vi "Begin.vi"(11 "Image Size":T1=enum."160x120") -> (0 "error out":errorcluster)   [LabVIEW 2012]
doc: "Called before other user functions, this VI is expected to open initial I/O refnums, load in file data, and do all program initialization. Notice that the <B>error out</B> terminal is simply used for data flow. Wiring it to other structures or subVIs ensures that this VI runs first."
uses:
  <vilib>/Rock Robotics/WPI/Camera/WPI_CameraImageSize.ctl
  <vilib>/Rock Robotics/WPI/Camera/WPI_CameraWhite Balance Values.ctl
  <vilib>/Rock Robotics/WPI/Camera/WPI_CameraExposure Values.ctl
  <vilib>/Rock Robotics/WPI/Camera/WPI_CameraFrameRate.ctl
  <vilib>/Rock Robotics/WPI/DriverStation/WPI_DriverStationRobotMode2.ctl
  <vilib>/Rock Robotics/SystemInterfaces/DIO/FPGA_DIOChannel.ctl
  <vilib>/Rock Robotics/SystemInterfaces/AI/FPGA_AIGyroChannel.ctl
  <vilib>/Rock Robotics/WPI/Relay/WPI_RelayDirection.ctl
  <vilib>/Rock Robotics/SystemInterfaces/DIO/FPGA_DIORelayChannel.ctl
  <vilib>/Rock Robotics/SystemInterfaces/DIO/FPGA_DIOPWMChannel.ctl
  <vilib>/Rock Robotics/SystemInterfaces/Typedef/FPGA_TypedefDigitalModule.ctl
  <vilib>/Rock Robotics/WPI/Joystick/WPI_JoystickDeviceEnum.ctl
  <vilib>/Rock Robotics/SystemInterfaces/AI/FPGA_AIChannel.ctl
  Robot Global Data.vi
  <vilib>/Rock Robotics/WPI/MotorControl/WPI_MotorControlOpen Victor.vi
  <vilib>/Rock Robotics/WPI/MotorControl/WPI_MotorControlOpen Jaguar.vi
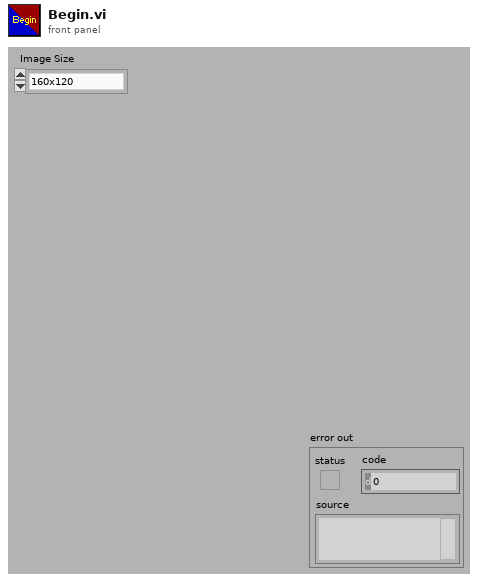
[diagram p1: front panel]
types:
  T1 = typedef "WPI_CameraImageSize.ctl" = enum16{"640x480", "320x240", "160x120"}
  T2 = typedef "FPGA_AIChannel.ctl" = enum8{"AI 1", "AI 2", "AI 3", "AI 4", "AI 5", "AI 6", "AI 7", "AI 8", "Invalid"}
  T3 = typedef "FPGA_TypedefDigitalModule.ctl" = enum16{"Digital Module 1", "Digital Module 2"}
  T4 = typedef "FPGA_DIOPWMChannel.ctl" = enum8{"PWM 1", "PWM 2", "PWM 3", "PWM 4", "PWM 5", "PWM 6", "PWM 7", "PWM 8", "PWM 9", "PWM 10", "Invalid"}
  T5 = typedef "WPI_JoystickDeviceEnum.ctl" = enum16{"USB 1", "USB 2", "USB 3", "USB 4", "Kinect 1", "Kinect 2"}
  T6 = typedef "FPGA_DIORelayChannel.ctl" = enum8{"Relay 1", "Relay 2", "Relay 3", "Relay 4", "Relay 5", "Relay 6", "Relay 7", "Relay 8", "Invalid"}
  T7 = typedef "WPI_RelayDirection.ctl" = enum16{"Both directions", "Forward only", "Reverse only"}
  T8 = typedef "FPGA_AIGyroChannel.ctl" = enum8{"AI 1", "AI 2", "Invalid"}
  T9 = typedef "FPGA_DIOChannel.ctl" = enum8{"DIO 1", "DIO 2", "DIO 3", "DIO 4", "DIO 5", "DIO 6", "DIO 7", "DIO 8", "DIO 9", "DIO 10", "DIO 11", "DIO 12", "DIO 13", "DIO 14", "Invalid"}
  T10 = typedef "WPI_DriverStationRobotMode2.ctl" = enum16{"Autonomous Disabled", "Autonomous Enabled", "Teleop Disabled", "Teleop Enabled", "Timeout", "Finish", "Test Disabled", "Test Enabled"}
  T11 = typedef "WPI_CameraFrameRate.ctl" = u32
  T12 = typedef "WPI_CameraExposure Values.ctl" = enum16{"Auto", "Flicker-free 50 Hz", "Flicker-free 60 Hz", "Hold current"}
  T13 = typedef "WPI_CameraWhite Balance Values.ctl" = enum16{"Auto", "Fixed indoor", "Fixed outdoor 1", "Fixed outdoor 2", "Fixed fluorescent 1", "Fixed fluorescent 2", "Hold current"}
  T14 = typedef "WPI_ServoDeviceRef.ctl" = cluster{"DeviceStatus":errorcluster, "Digital Module":T3, "PWM Channel":T4, "DeadBand":T15}
  T15 = typedef "WPI_PWMDeadband.ctl" = cluster{"Name":string, "maxPositivePwm":i32, "minPositivePwm":i32, "centerPwm":i32, "maxNegativePwm":i32, "minNegativePwm":i32, "angularRange":u16}
  T16 = typedef "WPI_CameraDevRef.ctl" = cluster{"Camera Address":string, "CameraStatus":errorcluster, "Acquire Image Notifier":refnum<notifier>}
  T17 = typedef "WPI_MotorControlDeviceRef.ctl" = cluster{"DeviceStatus":errorcluster, "Type":enum16{"PWM", "CAN"}, "PWM":cluster{"Digital Module":T3, "PWM Channel":T4, "DeadBand":T15}, "CAN":cluster{"Device Number":u8, "Control Mode":T18, "Semaphore":T19, "Max Vout":dbl}, "Invert":bool, "TransformRef":T20, "InvTransformRef":T20}
  T18 = typedef "WPI_CANJaguar_ControlMode.ctl" = enum8{"Percent VBus", "Current", "Speed", "Position", "Voltage"}
  T19 = typedef "Semaphore RefNum" = refnum<k1>
  T20 = typedef "WPI_PWMTransform_ConPane.ctl" = refnum<vi>
  T21 = typedef "WPI_JoystickDevRef.ctl" = cluster{"Device":T5}
  T22 = typedef "WPI_AnalogChannelDevRef.ctl" = cluster{"DevStatus":errorcluster, "Analog Module":T23, "Analog Channel":T2}
  T23 = typedef "FPGA_TypedefAnalogModule.ctl" = enum16{"Analog Module 1", "Analog Module 2"}
  T24 = typedef "WPI_RelayDevRef.ctl" = cluster{"DevStatus":errorcluster, "Relay Channel":T6, "Digital Module":T3, "Relay Direction":T7}
  T25 = typedef "WPI_DigitalInputDevRef.ctl" = cluster{"DevStatus":errorcluster, "DIO Channel":T9, "Digital Module":T3}
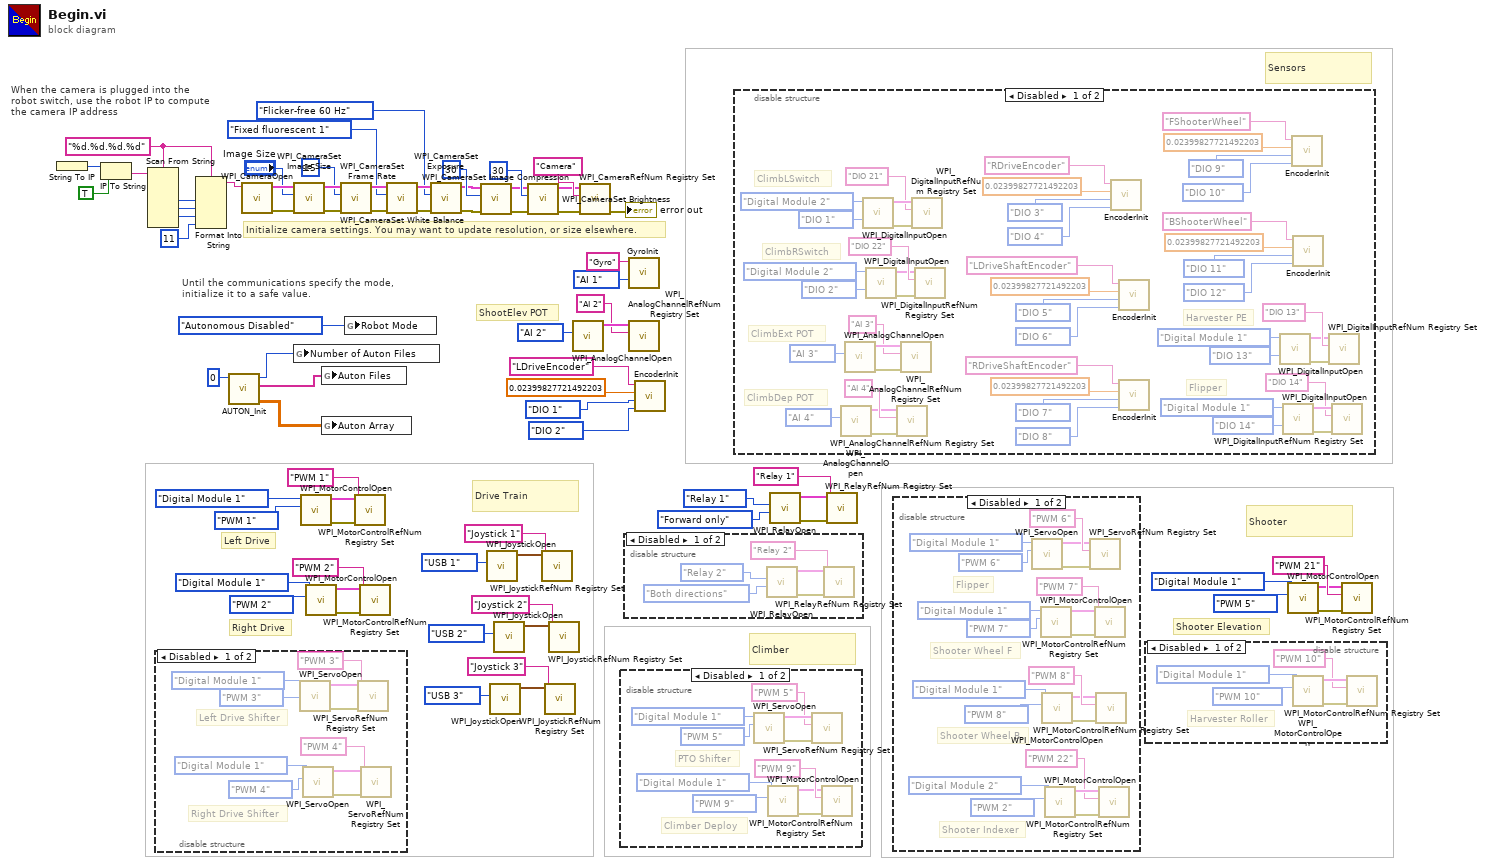
[diagram p0: block diagram]
diagram:
  w46 = "%d.%d.%d.%d" ("format string")
  # "ShootElev POT"
  # "Drive Train"
  # "Climber"
  # "Shooter"
  # "Shooter Elevation"
  # "Sensors"
  # "Right Drive"
  # "Left Drive"
  # "Until the communications specify the mode,\ninitialize it to a safe value."
  # "When the camera is plugged into the\nrobot switch, use the robot IP to compute\nthe camera IP address"
  # "Initialize camera settings. You may want to update resolution, or size elsewhere."
  n1 = String To IP() -> (0:w53:u32)  [unwired: 1 in]
  n2 = IP To String(1:TRUE ("dot notation? (F)"), 2:w53) -> (0:w51:string)
  n3 = Scan From String(format string=w46, input string=w51) -> (output 1=w50:i32, output 2=w49:i32, output 3=w48:i32)  [unwired: 7 in, 3 out]
  n4 = disable-structure shown="Disabled" {
    frame Disabled {
      # "Right Drive Shifter"
      # "Left Drive Shifter"
      n5 = call <vilib>:"WPI_ServoOpen.vi"("PWM Channel"=FPGA_DIOPWMChannel."PWM 3", "Digital Module (Module 1)"=FPGA_TypedefDigitalModule."Digital Module 1") -> ("error out"=w76:errorcluster, "ServoDeviceRef"=w77:T14)  [unwired: 8 in]
      n6 = call <vilib>:"WPI_ServoOpen.vi"("PWM Channel"=FPGA_DIOPWMChannel."PWM 4", "Digital Module (Module 1)"=FPGA_TypedefDigitalModule."Digital Module 1") -> ("error out"=w75:errorcluster, "ServoDeviceRef"=w82:T14)  [unwired: 8 in]
      n7 = call <vilib>:"WPI_ServoRefNum Registry Set.vi"("error in (no error)"=w76, "refnum name"="PWM 3", "ServoDeviceRef"=w77) -> ()  [unwired: 7 in, 2 out]
      n8 = call <vilib>:"WPI_ServoRefNum Registry Set.vi"("error in (no error)"=w75, "refnum name"="PWM 4", "ServoDeviceRef"=w82) -> ()  [unwired: 7 in, 2 out]
    }
    frame Enabled {
    }
  }
  n9 = Format Into String(format string=w46, w50, w49, w48, 11 ("Compression")) -> (resulting string=w44:string)  [unwired: 2 in, 1 out]
  n10 = call "AUTON_Init.vi"("Default File"=0) -> ("Auton Array"=w39:dbl[][], "Auton Files"=w40:string[], "Number of Auton Files"=w41:i64)  [unwired: 8 in]
  n11 = call <vilib>:"WPI_CameraOpen.vi"("Camera Address"=w44) -> ("error out"=w65:errorcluster, "CameraDevRef"=w66:T16)  [unwired: 1 in, 8 out]
  n12 = call <vilib>:"WPI_CameraSet Image Size.vi"("error in (no error)"=w65, "Image Size"="Image Size", "CameraDevRef"=w66) -> ("error out"=w64:errorcluster, "CameraDevRef Out"=w67:T16)  [unwired: 7 out]
  n13 = global write "Robot Global Data.vi" "Number of Auton Files"(w41) -> ()
  n14 = call-poly <vilib>:"WPI_MotorControlOpen.vi"("PWM Channel"=FPGA_DIOPWMChannel."PWM 1", "Digital Module (Module 1)"=FPGA_TypedefDigitalModule."Digital Module 1") -> ("error out"=w18:errorcluster, "MotorControlDeviceRef"=w19:T17)  [unwired: 8 in]
  n15 = call-poly <vilib>:"WPI_MotorControlOpen.vi"("PWM Channel"=FPGA_DIOPWMChannel."PWM 2", "Digital Module (Module 1)"=FPGA_TypedefDigitalModule."Digital Module 1") -> ("error out"=w25:errorcluster, "MotorControlDeviceRef"=w24:T17)  [unwired: 8 in]
  n16 = global write "Robot Global Data.vi" "Auton Files"(w40) -> ()
  n17 = global write "Robot Global Data.vi" "Auton Array"(w39) -> ()
  n18 = call <vilib>:"WPI_CameraSet Frame Rate.vi"("error in (no error)"=w64, "Frame Rate (fps)"=T11 15, "CameraDevRef"=w67) -> ("error out"=w63:errorcluster, "CameraDevRef Out"=w69:T16)  [unwired: 7 out]
  n19 = global write "Robot Global Data.vi" "Robot Mode"(WPI_DriverStationRobotMode2."Autonomous Disabled" ("Robot Mode")) -> ()
  n20 = call <vilib>:"WPI_MotorControlRefNum Registry Set.vi"("error in (no error)"=w18, "refnum name"="PWM 1", "MotorControlDevRef"=w19) -> ()  [unwired: 7 in, 2 out]
  n21 = call <vilib>:"WPI_MotorControlRefNum Registry Set.vi"("error in (no error)"=w25, "refnum name"="PWM 2", "MotorControlDevRef"=w24) -> ()  [unwired: 7 in, 2 out]
  n22 = call <vilib>:"WPI_CameraSet White Balance.vi"("error in (no error)"=w63, "White Balance"=WPI_CameraWhite_Balance_Values."Fixed fluorescent 1", "CameraDevRef"=w69) -> ("error out"=w62:errorcluster, "CameraDevRef Out"=w68:T16)  [unwired: 7 out]
  n23 = call <vilib>:"WPI_CameraSet Exposure.vi"("error in (no error)"=w62, "Exposure"=WPI_CameraExposure_Values."Flicker-free 60 Hz", "CameraDevRef"=w68) -> ("error out"=w61:errorcluster, "CameraDevRef Out"=w71:T16)  [unwired: 7 out]
  n24 = call <vilib>:"WPI_CameraSet Image Compression.vi"("error in (no error)"=w61, "Compression"=30, "CameraDevRef"=w71) -> ("error out"=w60:errorcluster, "CameraDevRef Out"=w70:T16)  [unwired: 7 out]
  n25 = call <vilib>:"WPI_JoystickOpen.vi"("JoystickDevice"=WPI_JoystickDeviceEnum."USB 1") -> ("JoystickDevRef"=w9:T21)  [unwired: 10 in]
  n26 = call <vilib>:"WPI_JoystickOpen.vi"("JoystickDevice"=WPI_JoystickDeviceEnum."USB 3") -> ("JoystickDevRef"=w15:T21)  [unwired: 10 in]
  n27 = call <vilib>:"WPI_JoystickOpen.vi"("JoystickDevice"=WPI_JoystickDeviceEnum."USB 2") -> ("JoystickDevRef"=w14:T21)  [unwired: 10 in]
  n28 = call <vilib>:"WPI_CameraSet Brightness.vi"("error in (no error)"=w60, "Brightness"=30, "CameraDevRef"=w70) -> ("error out"=w58:errorcluster, "CameraDevRef Out"=w59:T16)  [unwired: 7 out]
  n29 = call <vilib>:"WPI_JoystickRefNum Registry Set.vi"("refnum name"="Joystick 1", "JoystickDevRef"=w9) -> ()  [unwired: 8 in, 2 out]
  n30 = call <vilib>:"WPI_JoystickRefNum Registry Set.vi"("refnum name"="Joystick 3", "JoystickDevRef"=w15) -> ()  [unwired: 8 in, 2 out]
  n31 = call <vilib>:"WPI_JoystickRefNum Registry Set.vi"("refnum name"="Joystick 2", "JoystickDevRef"=w14) -> ()  [unwired: 8 in, 2 out]
  n32 = call <vilib>:"WPI_AnalogChannelOpen.vi"("Analog Channel"=FPGA_AIChannel."AI 2") -> ("AIDeviceRef"=w3:T22)  [unwired: 9 in, 1 out]
  n33 = call <vilib>:"WPI_CameraRefNum Registry Set.vi"("error in (no error)"=w58, "refnum name"="Camera", "CameraDevRef"=w59) -> ("error out"=→"error out":errorcluster)  [unwired: 8 out]
  n34 = disable-structure shown="Disabled" {
    frame Disabled {
      # "Climber Deploy"
      # "PTO Shifter"
      n35 = call <vilib>:"WPI_ServoOpen.vi"("PWM Channel"=FPGA_DIOPWMChannel."PWM 5", "Digital Module (Module 1)"=FPGA_TypedefDigitalModule."Digital Module 1") -> ("error out"=w94:errorcluster, "ServoDeviceRef"=w93:T14)  [unwired: 8 in]
      n36 = call-poly <vilib>:"WPI_MotorControlOpen.vi"("PWM Channel"=FPGA_DIOPWMChannel."PWM 9", "Digital Module (Module 1)"=FPGA_TypedefDigitalModule."Digital Module 1") -> ("error out"=w88:errorcluster, "MotorControlDeviceRef"=w87:T17)  [unwired: 8 in]
      n37 = call <vilib>:"WPI_ServoRefNum Registry Set.vi"("error in (no error)"=w94, "refnum name"="PWM 5", "ServoDeviceRef"=w93) -> ()  [unwired: 7 in, 2 out]
      n38 = call <vilib>:"WPI_MotorControlRefNum Registry Set.vi"("error in (no error)"=w88, "refnum name"="PWM 9", "MotorControlDevRef"=w87) -> ()  [unwired: 7 in, 2 out]
    }
    frame Enabled {
    }
  }
  n39 = disable-structure shown="Disabled" {
    frame Disabled {
      n40 = call <vilib>:"WPI_RelayOpen.vi"("Relay Direction"=WPI_RelayDirection."Both directions", "Relay Channel"=FPGA_DIORelayChannel."Relay 2") -> ("error out"=w95:errorcluster, "RelayDevRef"=w96:T24)  [unwired: 8 in]
      n41 = call <vilib>:"WPI_RelayRefNum Registry Set.vi"("error in (no error)"=w95, "refnum name"="Relay 2", "RelayDevRef"=w96) -> ()  [unwired: 7 in, 2 out]
    }
    frame Enabled {
    }
  }
  n42 = call "GyroInit.vi"("refnum name"="Gyro", "Analog Channel"=FPGA_AIGyroChannel."AI 1") -> ()  [unwired: 8 in]
  n43 = call <vilib>:"WPI_AnalogChannelRefNum Registry Set.vi"("refnum name"="AI 2", "AIDeviceRef"=w3) -> ()  [unwired: 8 in, 2 out]
  n44 = call "EncoderInit.vi"("refnum name"="LDriveEncoder", "DistancePerCount"=0.02399827721492203, "DIO Channel"=FPGA_DIOChannel."DIO 1", "DIO Channel 2"=FPGA_DIOChannel."DIO 2") -> ()  [unwired: 7 in]
  n45 = disable-structure shown="Disabled" {
    frame Disabled {
      # "ClimbRSwitch"
      # "ClimbLSwitch"
      # "ClimbDep POT"
      # "ClimbExt POT"
      # "Flipper"
      # "Harvester PE"
      n46 = call <vilib>:"WPI_AnalogChannelOpen.vi"("Analog Channel"=FPGA_AIChannel."AI 4") -> ("error out"=w114:errorcluster, "AIDeviceRef"=w115:T22)  [unwired: 9 in]
      n47 = call <vilib>:"WPI_AnalogChannelOpen.vi"("Analog Channel"=FPGA_AIChannel."AI 3") -> ("error out"=w113:errorcluster, "AIDeviceRef"=w112:T22)  [unwired: 9 in]
      n48 = call <vilib>:"WPI_DigitalInputOpen.vi"("DIO Channel"=FPGA_DIOChannel."DIO 1", "Digital Module (Module 1)"=FPGA_TypedefDigitalModule."Digital Module 2") -> ("error out"=w101:errorcluster, "DigitalInputDevRef"=w102:T25)  [unwired: 8 in]
      n49 = call <vilib>:"WPI_DigitalInputOpen.vi"("DIO Channel"=FPGA_DIOChannel."DIO 2", "Digital Module (Module 1)"=FPGA_TypedefDigitalModule."Digital Module 2") -> ("error out"=w108:errorcluster, "DigitalInputDevRef"=w107:T25)  [unwired: 8 in]
      n50 = call <vilib>:"WPI_AnalogChannelRefNum Registry Set.vi"("error in (no error)"=w114, "refnum name"="AI 4", "AIDeviceRef"=w115) -> ()  [unwired: 7 in, 2 out]
      n51 = call <vilib>:"WPI_AnalogChannelRefNum Registry Set.vi"("error in (no error)"=w113, "refnum name"="AI 3", "AIDeviceRef"=w112) -> ()  [unwired: 7 in, 2 out]
      n52 = call <vilib>:"WPI_DigitalInputRefNum Registry Set.vi"("error in (no error)"=w101, "refnum name"="DIO 21", "DigitalInputDevRef"=w102) -> ()  [unwired: 7 in, 2 out]
      n53 = call <vilib>:"WPI_DigitalInputRefNum Registry Set.vi"("error in (no error)"=w108, "refnum name"="DIO 22", "DigitalInputDevRef"=w107) -> ()  [unwired: 7 in, 2 out]
      n54 = call "EncoderInit.vi"("refnum name"="RDriveEncoder", "DistancePerCount"=0.02399827721492203, "DIO Channel"=FPGA_DIOChannel."DIO 3", "DIO Channel 2"=FPGA_DIOChannel."DIO 4") -> ()  [unwired: 7 in]
      n55 = call "EncoderInit.vi"("refnum name"="LDriveShaftEncoder", "DistancePerCount"=0.02399827721492203, "DIO Channel"=FPGA_DIOChannel."DIO 5", "DIO Channel 2"=FPGA_DIOChannel."DIO 6") -> ()  [unwired: 7 in]
      n56 = call "EncoderInit.vi"("refnum name"="RDriveShaftEncoder", "DistancePerCount"=0.02399827721492203, "DIO Channel"=FPGA_DIOChannel."DIO 7", "DIO Channel 2"=FPGA_DIOChannel."DIO 8") -> ()  [unwired: 7 in]
      n57 = call <vilib>:"WPI_DigitalInputOpen.vi"("DIO Channel"=FPGA_DIOChannel."DIO 13", "Digital Module (Module 1)"=FPGA_TypedefDigitalModule."Digital Module 1") -> ("error out"=w126:errorcluster, "DigitalInputDevRef"=w125:T25)  [unwired: 8 in]
      n58 = call <vilib>:"WPI_DigitalInputOpen.vi"("DIO Channel"=FPGA_DIOChannel."DIO 14", "Digital Module (Module 1)"=FPGA_TypedefDigitalModule."Digital Module 1") -> ("error out"=w119:errorcluster, "DigitalInputDevRef"=w120:T25)  [unwired: 8 in]
      n59 = call "EncoderInit.vi"("refnum name"="FShooterWheel", "DistancePerCount"=0.02399827721492203, "DIO Channel"=FPGA_DIOChannel."DIO 9", "DIO Channel 2"=FPGA_DIOChannel."DIO 10") -> ()  [unwired: 7 in]
      n60 = call "EncoderInit.vi"("refnum name"="BShooterWheel", "DistancePerCount"=0.02399827721492203, "DIO Channel"=FPGA_DIOChannel."DIO 11", "DIO Channel 2"=FPGA_DIOChannel."DIO 12") -> ()  [unwired: 7 in]
      n61 = call <vilib>:"WPI_DigitalInputRefNum Registry Set.vi"("error in (no error)"=w126, "refnum name"="DIO 13", "DigitalInputDevRef"=w125) -> ()  [unwired: 7 in, 2 out]
      n62 = call <vilib>:"WPI_DigitalInputRefNum Registry Set.vi"("error in (no error)"=w119, "refnum name"="DIO 14", "DigitalInputDevRef"=w120) -> ()  [unwired: 7 in, 2 out]
    }
    frame Enabled {
    }
  }
  n63 = call <vilib>:"WPI_RelayOpen.vi"("Relay Direction"=WPI_RelayDirection."Forward only", "Relay Channel"=FPGA_DIORelayChannel."Relay 1") -> ("error out"=w32:errorcluster, "RelayDevRef"=w31:T24)  [unwired: 8 in]
  n64 = call <vilib>:"WPI_RelayRefNum Registry Set.vi"("error in (no error)"=w32, "refnum name"="Relay 1", "RelayDevRef"=w31) -> ()  [unwired: 7 in, 2 out]
  n65 = disable-structure shown="Disabled" {
    frame Disabled {
      # "Shooter Wheel B"
      # "Flipper"
      # "Shooter Indexer"
      # "Shooter Wheel F"
      n66 = call <vilib>:"WPI_ServoOpen.vi"("PWM Channel"=FPGA_DIOPWMChannel."PWM 6", "Digital Module (Module 1)"=FPGA_TypedefDigitalModule."Digital Module 1") -> ("error out"=w153:errorcluster, "ServoDeviceRef"=w154:T14)  [unwired: 8 in]
      n67 = call-poly <vilib>:"WPI_MotorControlOpen.vi"("PWM Channel"=FPGA_DIOPWMChannel."PWM 7", "Digital Module (Module 1)"=FPGA_TypedefDigitalModule."Digital Module 1") -> ("error out"=w164:errorcluster, "MotorControlDeviceRef"=w165:T17)  [unwired: 8 in]
      n68 = call-poly <vilib>:"WPI_MotorControlOpen.vi"("PWM Channel"=FPGA_DIOPWMChannel."PWM 8", "Digital Module (Module 1)"=FPGA_TypedefDigitalModule."Digital Module 1") -> ("error out"=w150:errorcluster, "MotorControlDeviceRef"=w149:T17)  [unwired: 8 in]
      n69 = call-poly <vilib>:"WPI_MotorControlOpen.vi"("PWM Channel"=FPGA_DIOPWMChannel."PWM 2", "Digital Module (Module 1)"=FPGA_TypedefDigitalModule."Digital Module 2") -> ("error out"=w160:errorcluster, "MotorControlDeviceRef"=w161:T17)  [unwired: 8 in]
      n70 = call <vilib>:"WPI_ServoRefNum Registry Set.vi"("error in (no error)"=w153, "refnum name"="PWM 6", "ServoDeviceRef"=w154) -> ()  [unwired: 7 in, 2 out]
      n71 = call <vilib>:"WPI_MotorControlRefNum Registry Set.vi"("error in (no error)"=w164, "refnum name"="PWM 7", "MotorControlDevRef"=w165) -> ()  [unwired: 7 in, 2 out]
      n72 = call <vilib>:"WPI_MotorControlRefNum Registry Set.vi"("error in (no error)"=w150, "refnum name"="PWM 8", "MotorControlDevRef"=w149) -> ()  [unwired: 7 in, 2 out]
      n73 = call <vilib>:"WPI_MotorControlRefNum Registry Set.vi"("error in (no error)"=w160, "refnum name"="PWM 22", "MotorControlDevRef"=w161) -> ()  [unwired: 7 in, 2 out]
    }
    frame Enabled {
    }
  }
  n74 = disable-structure shown="Disabled" {
    frame Disabled {
      # "Harvester Roller"
      n75 = call-poly <vilib>:"WPI_MotorControlOpen.vi"("PWM Channel"=FPGA_DIOPWMChannel."PWM 10", "Digital Module (Module 1)"=FPGA_TypedefDigitalModule."Digital Module 1") -> ("error out"=w170:errorcluster, "MotorControlDeviceRef"=w171:T17)  [unwired: 8 in]
      n76 = call <vilib>:"WPI_MotorControlRefNum Registry Set.vi"("error in (no error)"=w170, "refnum name"="PWM 10", "MotorControlDevRef"=w171) -> ()  [unwired: 7 in, 2 out]
    }
    frame Enabled {
    }
  }
  n77 = call-poly <vilib>:"WPI_MotorControlOpen.vi"("PWM Channel"=FPGA_DIOPWMChannel."PWM 5", "Digital Module (Module 1)"=FPGA_TypedefDigitalModule."Digital Module 1") -> ("error out"=w6:errorcluster, "MotorControlDeviceRef"=w5:T17)  [unwired: 8 in]
  n78 = call <vilib>:"WPI_MotorControlRefNum Registry Set.vi"("error in (no error)"=w6, "refnum name"="PWM 21", "MotorControlDevRef"=w5) -> ()  [unwired: 7 in, 2 out]
